vi "Mapping Error Handler (Multiple).vi"(8 "error in (no error)":errorcluster, 11 "Mapping Errors":T1[](array[typedef])) -> (0 "error out":errorcluster, 3 "Continue?":bool)   [LabVIEW 2016, in "System Mapping Tool.lvlib"]
uses:
  System Mapping Tool.lvlib
  TypeDefs/Mapping Error Cluster.ctl
  TypeDefs/Mapping Error.ctl
  TypeDefs/Mapping Error Groups.ctl
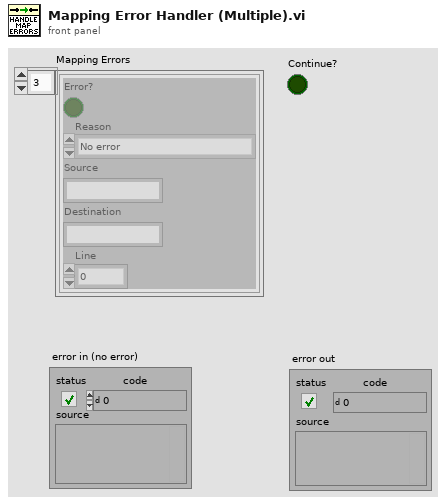
[diagram p1: front panel]
types:
  T1 = typedef "System Mapping Tool.lvlib/Mapping Error Cluster.ctl" = cluster{"Error?":bool, "Reason":T2, "Source":string, "Destination":string, "Line":i32}
  T2 = typedef "System Mapping Tool.lvlib/Mapping Error.ctl" = enum16{"No error", "Channels already mapped", "Source is not valid", "Destination is not valid", "Destination already mapped", "Destination mapped twice"}
  T3 = typedef "System Mapping Tool.lvlib/Mapping Error Groups.ctl" = cluster{"Mapping Errors":string[][], "Duplicate Mappings":string[][], "Mappings to Import":string[][]}
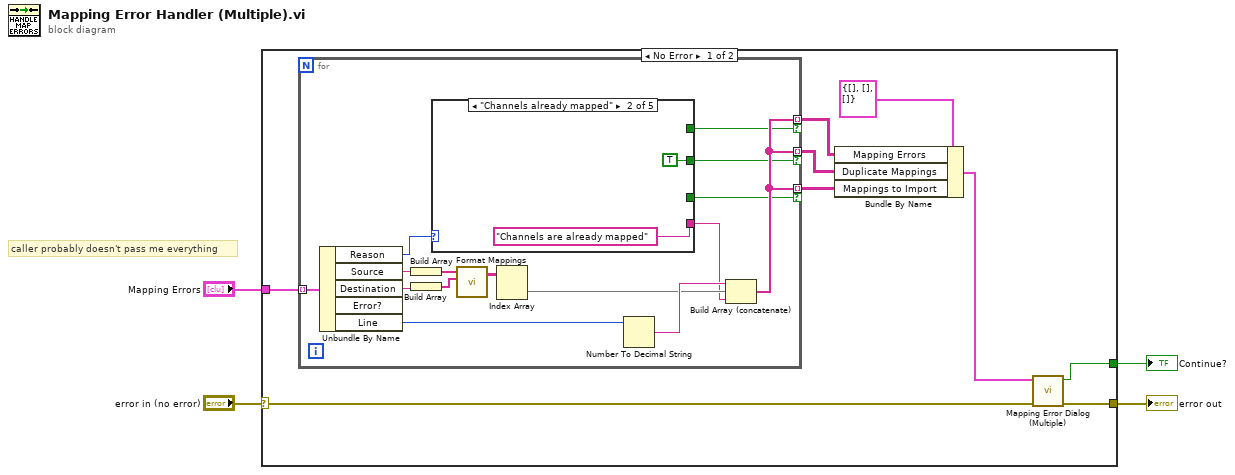
[diagram p0: block diagram]
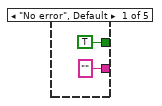
[diagram p2: hidden frame]
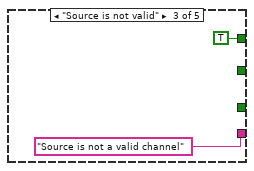
[diagram p3: hidden frame]
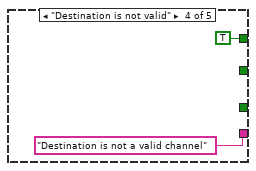
[diagram p4: hidden frame]
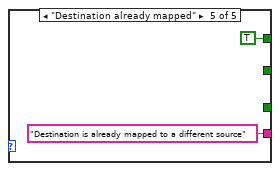
[diagram p5: hidden frame]
diagram:
  # "caller probably doesn't pass me everything"
  n1 = case shown="No Error" "error in (no error)" {
    selector: "error in (no error)" -> [w12 w39]
    tunnel: [w11 w39] -> w3
    tunnel: "Mapping Errors" -> [w13 _]
    tunnel: [w10 _] -> w1
    frame No Error {
      n2 = for {
        tunnel: w13 -> [w28] mode=indexing
        tunnel: [w17] -> w6 mode=indexing if=w16
        tunnel: [w17] -> w7 mode=indexing if=w15
        tunnel: [w17] -> w8 mode=indexing if=w14
        n3 = Unbundle By Name(w28) -> ("Reason"=w27:T2, "Source"=w26:string, "Destination"=w23:string, "Line"=w25:i32)  [unwired: 1 out]
        n4 = Build Array(w26) -> (w24:string[])
        n5 = Build Array(w23) -> (w22:string[])
        n6 = case shown="\"Channels already mapped\"" w27 {
          tunnel: ["" "Channels are already mapped" "Source is not a valid channel" "Destination is not a valid channel" "Destination is already mapped to a different source"] -> w18
          tunnel: [_ _ TRUE TRUE TRUE] -> w16
          tunnel: [_ TRUE _ _ _] -> w15
          tunnel: [TRUE _ _ _ _] -> w14
          frame "No error", Default {
          }
          frame "Channels already mapped" {
          }
          frame "Source is not valid" {
          }
          frame "Destination is not valid" {
          }
          frame "Destination already mapped" {
          }
        }
        n7 = call "Format Mappings.vi"("Destinations"=w22, "Sources"=w24) -> ("Mappings"=w21:string[][])  [unwired: 3 in]
        n8 = Index Array(array=w21) -> (element=w19:string[])  [unwired: 2 in]
        n9 = Number To Decimal String(number=w25) -> (decimal integer string=w20:string)  [unwired: 1 in]
        n10 = Build Array (concatenate)(w20, w19, w18) -> (w17:string[])
      }
      n11 = Bundle By Name(cluster=T3 {"Mapping Errors"=[], "Duplicate Mappings"=[], "Mappings to Import"=[]} ("Mapping Types"), "Mapping Errors"=w6, "Duplicate Mappings"=w7, "Mappings to Import"=w8) -> (w5:T3)
      n12 = call "Mapping Error Dialog (Multiple).vi"("error in (no error)"=w12, "Mapping Types"=w5) -> ("error out"=w11:errorcluster, "Continue?"=w10:bool)  [unwired: 8 in]
    }
    frame Error {
    }
  }
  "error out" <- w3
  "Continue?" <- w1
